vi "Autonomous Independent.vi"   [LabVIEW 2013]
doc: "This VI is called when autonomous begins, and will automatically be terminated when autonomous ends. You can carry out timed or sensor driven robot movement independently without needing to return to the caller."
uses:
  <vilib>/Rock Robotics/WPI/SafetyOutput/WPI_SafetyOutputConfigMenu.ctl
  <vilib>/Rock Robotics/WPI/Solenoid/WPI_SolenoidValue.ctl
  <vilib>/Rock Robotics/WPI/Relay/WPI_RelayValue.ctl
  Robot Global Data.vi
  <vilib>/Rock Robotics/WPI/RobotDrive/WPI_RobotDriveGetSetRefNum.vi
  <vilib>/Rock Robotics/WPI/Solenoid/WPI_SolenoidSetEnum.vi
  <vilib>/Rock Robotics/WPI/RobotDrive/WPI_RobotDriveArcadeDrive_Standard(NoSaturation).vi
  <vilib>/Rock Robotics/WPI/Joystick/WPI_JoystickGetSetRefNum.vi
panel:
  # "Be sure to right-click and choose Data Operations>>Make Current Value default if you want to save the array values with the VI"
types:
  T1 = typedef "WPI_SafetyOutputConfigMenu.ctl" = enum16{"Enable", "Disable"}
  T2 = typedef "WPI_RelayValue.ctl" = enum16{"Off", "On", "Forward", "Reverse"}
  T3 = typedef "WPI_SolenoidValue.ctl" = enum16{"Off", "On", "Forward", "Reverse"}
  T4 = typedef "WPI_JoystickDevRef.ctl" = cluster{"Device":T5}
  T5 = typedef "WPI_JoystickDeviceEnum.ctl" = enum16{"USB 1", "USB 2", "USB 3", "USB 4", "Kinect 1", "Kinect 2"}
  T6 = cluster{"axis 1 (x)":dbl, "axis 2 (y)":dbl, "axis 3 (throttle)":dbl, "axis 4":dbl, "axis 5":dbl, "axis 6":dbl}
  T7 = typedef "WPI_RobotDriveDevRef.ctl" = cluster{"DevStatus":errorcluster, "Motors[]":T8[], "Square Inputs":bool, "Max Output":dbl, "Isochronous":bool}
  T8 = typedef "WPI_MotorControlDeviceRef.ctl" = cluster{"DeviceStatus":errorcluster, "Type":enum16{"PWM", "CAN"}, "PWM":cluster{"Digital Module":T9, "PWM Channel":T10, "DeadBand":T11}, "CAN":cluster{"Device Number":u8, "Control Mode":T12, "Semaphore":T13, "Max Vout":dbl}, "Invert":bool, "TransformRef":T14, "InvTransformRef":T14}
  T9 = typedef "FPGA_TypedefDigitalModule.ctl" = enum16{"Digital Module 1", "Digital Module 2"}
  T10 = typedef "FPGA_DIOPWMChannel.ctl" = enum8{"PWM 1", "PWM 2", "PWM 3", "PWM 4", "PWM 5", "PWM 6", "PWM 7", "PWM 8", "PWM 9", "PWM 10", "Invalid"}
  T11 = typedef "WPI_PWMDeadband.ctl" = cluster{"Name":string, "maxPositivePwm":i32, "minPositivePwm":i32, "centerPwm":i32, "maxNegativePwm":i32, "minNegativePwm":i32, "angularRange":u16}
  T12 = typedef "WPI_CANJaguar_ControlMode.ctl" = enum8{"Percent VBus", "Current", "Speed", "Position", "Voltage"}
  T13 = typedef "Semaphore RefNum" = refnum<k1>
  T14 = typedef "WPI_PWMTransform_ConPane.ctl" = refnum<vi>
  T15 = typedef "WPI_SolenoidDevRef.ctl" = cluster{"DevStatus":errorcluster, "Solenoid Module":T16, "Forward Solenoid Channel":T17, "Reverse Solenoid Channel":T17}
  T16 = typedef "FPGA_TypedefSolenoidModule.ctl" = enum16{"Solenoid Module 1", "Solenoid Module 2"}
  T17 = typedef "WPI_SolenoidChannel.ctl" = enum8{"Solenoid 1", "Solenoid 2", "Solenoid 3", "Solenoid 4", "Solenoid 5", "Solenoid 6", "Solenoid 7", "Solenoid 8", "Invalid"}
  T18 = typedef "WPI_RelayDevRef.ctl" = cluster{"DevStatus":errorcluster, "Relay Channel":T19, "Digital Module":T9, "Relay Direction":T20}
  T19 = typedef "FPGA_DIORelayChannel.ctl" = enum8{"Relay 1", "Relay 2", "Relay 3", "Relay 4", "Relay 5", "Relay 6", "Relay 7", "Relay 8", "Invalid"}
  T20 = typedef "WPI_RelayDirection.ctl" = enum16{"Both directions", "Forward only", "Reverse only"}
  T21 = typedef "WPI_AnalogChannelDevRef.ctl" = cluster{"DevStatus":errorcluster, "Analog Module":T22, "Analog Channel":T23}
  T22 = typedef "FPGA_TypedefAnalogModule.ctl" = enum16{"Analog Module 1", "Analog Module 2"}
  T23 = typedef "FPGA_AIChannel.ctl" = enum8{"AI 1", "AI 2", "AI 3", "AI 4", "AI 5", "AI 6", "AI 7", "AI 8", "Invalid"}
diagram:
  (unwired) "This code sets the toggle rate used by the Periodic Tasks VI.  For autonomous mode we slowly flash the USER1 LED on the cRIO.  Look at the Periodic Tasks VI to see how this global value is used."
  (unwired) "Autonomous sample code is disabled so your robot doesn't unexpectantly run in Autonomous mode.  To enable this code, right-click on the edge of the frame and choose either \"Remove Diagram Disable Structure\" or \"Enable This Subdiagram\". You should only enable one of the samples."
  (unwired) "This function is run in parallel when the autonomous period begins. It will be terminated automatically when the period ends.\n\nNote that all Driver Station inputs are automatically latched and will not change once auto begins."
  # "This tells you the driver position\nand alliance color"
  n1 = call <vilib>:"WPI_DriverStationGet Digital Input.vi"() -> ("Driver Station Digital Input (1-8)"=w4:bool[])  [unwired: 11 out]
  n2 = while {
    stop <- FALSE stop-if-true
    n3 = call <vilib>:"WPI_DriverStationReport Robot Code State.vi"("Autonomous"=TRUE) -> ()  [unwired: 10 in, 1 out]
    n4 = Wait (ms)(milliseconds to wait=u32 20) -> ()  [unwired: 1 out]
  }
  n5 = call <vilib>:"WPI_DriverStationGet Alliance Info.vi"() -> ()  [unwired: 12 out]
  n6 = call <vilib>:"WPI_DriverStationGet Analog Input.vi"() -> ()  [unwired: 12 out]
  n7 = global write "Robot Global Data.vi" "LED toggle rate (ms)"(u32 500 ("LED ms toggle rate")) -> ()
  n8 = Index Array(array=w4) -> (element #1=w2:bool, element #2=w1:bool)  [unwired: 8 in, 6 out]
  n9 = case shown="True" w2 {
    frame False {
    }
    frame True {
      # "Every 20ms, report that we are running autonomous\ncode. Loop will abort the same time as the VI."
      # "Use time and/or sensors to control how the robot drives."
      n10 = call <vilib>:"WPI_JoystickRefNum Registry Get.vi"("refnum name"="Joystick 1") -> ("JoystickDevRef"=w35:T4)  [unwired: 1 in, 9 out]
      n11 = call <vilib>:"WPI_JoystickGet.vi"("JoystickDevRef"=w35) -> ("Axes"=w33:T6)  [unwired: 1 in, 5 out]
      n12 = Unbundle By Name(w33) -> ()  [unwired: 1 out]
      n13 = Cluster To Array(cluster=w33) -> (array=w34:dbl[])
      n14 = call <vilib>:"WPI_RobotDriveRefNum Registry Get.vi"("refnum name"="Left and Right Motors") -> ("error out"=w30:errorcluster, "RobotDriveDevRef"=w29:T7)  [unwired: 9 in]
      n15 = call <vilib>:"SD Write Numeric Array.vi"("Numeric Array"=w34, "Name"="Joystick 1/Axes") -> ()  [unwired: 8 in, 2 out]
      n16 = call <vilib>:"WPI_RobotDriveSafetyConfig.vi"("error in (no error)"=w30, "mode"=WPI_SafetyOutputConfigMenu."Disable", "RobotDriveDevRef"=w29) -> ("error out"=w14:errorcluster, "RobotDriveDevRef"=w15:T7)  [unwired: 7 in]
      n17 = call <vilib>:"WPI_SolenoidRefNum Registry Get.vi"("refnum name"="clamp") -> ("error out"=w18:errorcluster, "SolenoidDevRef"=w19:T15)  [unwired: 9 in]
      n18 = call <vilib>:"WPI_SolenoidRefNum Registry Get.vi"("refnum name"="pickup") -> ("error out"=w16:errorcluster, "SolenoidDevRef"=w17:T15)  [unwired: 9 in]
      n19 = call <vilib>:"WPI_SolenoidRefNum Registry Get.vi"("refnum name"="gear") -> ("error out"=w20:errorcluster, "SolenoidDevRef"=w21:T15)  [unwired: 9 in]
      n20 = call <vilib>:"WPI_SolenoidRefNum Registry Get.vi"("refnum name"="lock") -> ("error out"=w22:errorcluster, "SolenoidDevRef"=w23:T15)  [unwired: 9 in]
      n21 = call <vilib>:"WPI_RelayRefNum Registry Get.vi"("refnum name"="light") -> ("error out"=w8:errorcluster, "RelayDevRef"=w9:T18)  [unwired: 9 in]
      n22 = flat-sequence {
        tunnel: [w123] -> w104
        tunnel: [w122] -> w103
        tunnel: [w121] -> w102
        tunnel: [w120] -> w101
        tunnel: [w119] -> w100
        tunnel: [w118] -> w99
        tunnel: [w117] -> w98
        tunnel: [w116] -> w97
        tunnel: [w115] -> w96
        tunnel: [w114] -> w95
        tunnel: w8 -> [w106]
        tunnel: w9 -> [w107]
        tunnel: w14 -> [w122]
        tunnel: w15 -> [w123]
        tunnel: w16 -> [w124]
        tunnel: w17 -> [w125]
        tunnel: w18 -> [w126]
        tunnel: w19 -> [w127]
        tunnel: w20 -> [w108]
        tunnel: w21 -> [w109]
        tunnel: w22 -> [w110]
        tunnel: w23 -> [w111]
        tunnel: [w139] -> w94
        tunnel: w104 -> [w139]
        tunnel: w103 -> [w138]
        tunnel: [w138] -> w93
        tunnel: w102 -> [w137]
        tunnel: [w137] -> w92
        tunnel: [w136] -> w91
        tunnel: w101 -> [w136]
        tunnel: w100 -> [w135]
        tunnel: [w135] -> w90
        tunnel: [w134] -> w89
        tunnel: w99 -> [w134]
        tunnel: [w133] -> w88
        tunnel: w98 -> [w133]
        tunnel: [w132] -> w87
        tunnel: w97 -> [w132]
        tunnel: [w131] -> w86
        tunnel: w96 -> [w131]
        tunnel: [w130] -> w85
        tunnel: w95 -> [w130]
        tunnel: w94 -> [w154]
        tunnel: w93 -> [w153]
        tunnel: w92 -> [w150]
        tunnel: [w150] -> w84
        tunnel: [w149] -> w83
        tunnel: w91 -> [w149]
        tunnel: w90 -> [w148]
        tunnel: [w148] -> w82
        tunnel: [w147] -> w81
        tunnel: w89 -> [w147]
        tunnel: [w146] -> w80
        tunnel: [w145] -> w79
        tunnel: [w144] -> w78
        tunnel: w88 -> [w144]
        tunnel: [w143] -> w77
        tunnel: w87 -> [w143]
        tunnel: [w142] -> w76
        tunnel: w86 -> [w142]
        tunnel: [w141] -> w75
        tunnel: w85 -> [w141]
        tunnel: w13 -> [w166]
        tunnel: w12 -> [w165]
        tunnel: w84 -> [w164]
        tunnel: [w164] -> w74
        tunnel: [w163] -> w73
        tunnel: w83 -> [w163]
        tunnel: w82 -> [w162]
        tunnel: [w162] -> w72
        tunnel: [w161] -> w71
        tunnel: w81 -> [w161]
        tunnel: w80 -> [w160]
        tunnel: [w160] -> w70
        tunnel: w79 -> [w159]
        tunnel: [w159] -> w69
        tunnel: [w158] -> w68
        tunnel: w78 -> [w158]
        tunnel: [w157] -> w67
        tunnel: w77 -> [w157]
        tunnel: [w156] -> w66
        tunnel: w76 -> [w156]
        tunnel: [w155] -> w65
        tunnel: w75 -> [w155]
        tunnel: w74 -> [w180]
        tunnel: w73 -> [w179]
        tunnel: w72 -> [w186]
        tunnel: [w186] -> w64
        tunnel: [w185] -> w63
        tunnel: w71 -> [w185]
        tunnel: w70 -> [w184]
        tunnel: w69 -> [w183]
        tunnel: [w180] -> w62
        tunnel: [w179] -> w61
        tunnel: [w178] -> w60
        tunnel: w68 -> [w178]
        tunnel: [w177] -> w59
        tunnel: w67 -> [w177]
        tunnel: [w176] -> w58
        tunnel: w66 -> [w176]
        tunnel: [w175] -> w57
        tunnel: w65 -> [w175]
        tunnel: w64 -> [w195]
        tunnel: [w195] -> w56
        tunnel: w63 -> [w194]
        tunnel: [w194] -> w55
        tunnel: w62 -> [w193]
        tunnel: [w193] -> w54
        tunnel: w61 -> [w192]
        tunnel: [w192] -> w53
        tunnel: w60 -> [w191]
        tunnel: [w191] -> w52
        tunnel: w59 -> [w190]
        tunnel: [w190] -> w51
        tunnel: w58 -> [w189]
        tunnel: [w189] -> w50
        tunnel: w57 -> [w188]
        tunnel: [w188] -> w49
        tunnel: w56 -> [w205]
        tunnel: [w205] -> w48
        tunnel: w55 -> [w204]
        tunnel: [w204] -> w47
        tunnel: w54 -> [w203]
        tunnel: [w203] -> w46
        tunnel: w53 -> [w202]
        tunnel: [w202] -> w45
        tunnel: w52 -> [w201]
        tunnel: w51 -> [w200]
        tunnel: w50 -> [w197]
        tunnel: w49 -> [w196]
        tunnel: w48 -> [w209]
        tunnel: [w209] -> w44
        tunnel: w47 -> [w208]
        tunnel: [w208] -> w43
        tunnel: w46 -> [w207]
        tunnel: [w207] -> w42
        tunnel: w45 -> [w206]
        tunnel: [w206] -> w41
        tunnel: w44 -> [w217]
        tunnel: [w217] -> w40
        tunnel: w43 -> [w216]
        tunnel: [w216] -> w39
        tunnel: w42 -> [w214]
        tunnel: w41 -> [w213]
        tunnel: w40 -> [w219]
        tunnel: [w219] -> w37
        tunnel: [w218] -> w38
        tunnel: w39 -> [w218]
        tunnel: w38 -> [w221]
        tunnel: w37 -> [w222]
        frame #0 {
          n23 = call-poly <vilib>:"WPI_SolenoidSet.vi"("error in (no error)"=w126, "Value"=WPI_SolenoidValue."Reverse", "SolenoidDevRef"=w127) -> ("error out"=w114:errorcluster, "SolenoidDevRef"=w115:T15)  [unwired: 7 in]
          n24 = call-poly <vilib>:"WPI_SolenoidSet.vi"("error in (no error)"=w108, "Value"=WPI_SolenoidValue."Forward", "SolenoidDevRef"=w109) -> ("error out"=w118:errorcluster, "SolenoidDevRef"=w119:T15)  [unwired: 7 in]
          n25 = call-poly <vilib>:"WPI_SolenoidSet.vi"("error in (no error)"=w110, "Value"=WPI_SolenoidValue."Forward", "SolenoidDevRef"=w111) -> ("error out"=w120:errorcluster, "SolenoidDevRef"=w121:T15)  [unwired: 7 in]
          n26 = call-poly <vilib>:"WPI_SolenoidSet.vi"("error in (no error)"=w124, "Value"=WPI_SolenoidValue."Reverse", "SolenoidDevRef"=w125) -> ("error out"=w116:errorcluster, "SolenoidDevRef"=w117:T15)  [unwired: 7 in]
          n27 = call <vilib>:"WPI_RelaySet.vi"("error in (no error)"=w106, "RelayValue"=WPI_RelayValue."Forward", "RelayDevRef"=w107) -> ()  [unwired: 7 in, 2 out]
        }
        frame #1 {
          n28 = Wait (ms)(milliseconds to wait=u32 400) -> ()  [unwired: 1 out]
        }
        frame #2 {
          n29 = call-poly <vilib>:"WPI_RobotDriveArcadeDrive.vi"("error in (no error)"=w153, "Y axis value"=0.8, "X axis value"=0.0, "RobotDriveDevRef"=w154) -> ("error out"=w145:errorcluster, "RobotDriveDevRef"=w146:T7)  [unwired: 5 in, 1 out]
        }
        frame #3 {
          n30 = while {
            tunnel: w166 -> [w174]
            tunnel: w165 -> [w173]
            stop <- w171 stop-if-true
            n31 = call <vilib>:"WPI_AnalogChannelGetVoltage.vi"("error in (no error)"=w173, "AIDeviceRef"=w174) -> ("Voltage"=w169:dbl)  [unwired: 7 in, 2 out]
            n32 = Wait (ms)(milliseconds to wait=u32 10) -> ()  [unwired: 1 out]
            n33 = Divide(x=w169, y=0.12) -> (x/y=w170:dbl)
            n34 = Less?(x=w170, y=7.0) -> (x < y?=w171:bool)
          }
        }
        frame #4 {
          # "stop"
          n35 = call-poly <vilib>:"WPI_RobotDriveArcadeDrive.vi"("error in (no error)"=w183, "Y axis value"=0.0, "X axis value"=0.0, "RobotDriveDevRef"=w184) -> ()  [unwired: 5 in, 3 out]
        }
        frame #5 {
          n36 = Wait (ms)(milliseconds to wait=u32 500) -> ()  [unwired: 1 out]
        }
        frame #6 {
          # "let go of ball"
          n37 = call-poly <vilib>:"WPI_SolenoidSet.vi"("error in (no error)"=w196, "Value"=WPI_SolenoidValue."Forward", "SolenoidDevRef"=w197) -> ()  [unwired: 7 in, 2 out]
          n38 = call-poly <vilib>:"WPI_SolenoidSet.vi"("error in (no error)"=w200, "Value"=WPI_SolenoidValue."Forward", "SolenoidDevRef"=w201) -> ()  [unwired: 7 in, 2 out]
        }
        frame #7 {
          # "check for hot goal"
          n39 = while {
            stop <- w212 stop-if-true
            n40 = Wait (ms)(milliseconds to wait=u32 10) -> ()  [unwired: 1 out]
            n41 = call <vilib>:"SD Read Boolean.vi"("Name"="Goal is hot") -> ("Boolean"=w212:bool)  [unwired: 8 in, 2 out]
          }
        }
        frame #8 {
          # "fire"
          n42 = call-poly <vilib>:"WPI_SolenoidSet.vi"("error in (no error)"=w213, "Value"=WPI_SolenoidValue."Reverse", "SolenoidDevRef"=w214) -> ()  [unwired: 7 in, 2 out]
        }
        frame #9 {
          n43 = Wait (ms)(milliseconds to wait=u32 2000) -> ()  [unwired: 1 out]
        }
        frame #10 {
          # "ready for tele"
          n44 = call-poly <vilib>:"WPI_SolenoidSet.vi"("error in (no error)"=w221, "Value"=WPI_SolenoidValue."Reverse", "SolenoidDevRef"=w222) -> ()  [unwired: 7 in, 2 out]
        }
      }
      n45 = call <vilib>:"WPI_AnalogChannelRefNum Registry Get.vi"("refnum name"="sensor") -> ("error out"=w12:errorcluster, "AIDeviceRef"=w13:T21)  [unwired: 9 in]
    }
  }
  n46 = case shown="True" w1 {
    frame False {
    }
    frame True {
      n47 = call <vilib>:"WPI_RobotDriveRefNum Registry Get.vi"("refnum name"="Left and Right Motors") -> ("error out"=w311:errorcluster, "RobotDriveDevRef"=w310:T7)  [unwired: 9 in]
      n48 = call <vilib>:"WPI_RobotDriveSafetyConfig.vi"("error in (no error)"=w311, "mode"=WPI_SafetyOutputConfigMenu."Disable", "RobotDriveDevRef"=w310) -> ("error out"=w293:errorcluster, "RobotDriveDevRef"=w294:T7)  [unwired: 7 in]
      n49 = call <vilib>:"WPI_SolenoidRefNum Registry Get.vi"("refnum name"="clamp") -> ("error out"=w299:errorcluster, "SolenoidDevRef"=w300:T15)  [unwired: 9 in]
      n50 = call <vilib>:"WPI_SolenoidRefNum Registry Get.vi"("refnum name"="pickup") -> ("error out"=w297:errorcluster, "SolenoidDevRef"=w298:T15)  [unwired: 9 in]
      n51 = call <vilib>:"WPI_SolenoidRefNum Registry Get.vi"("refnum name"="gear") -> ("error out"=w301:errorcluster, "SolenoidDevRef"=w302:T15)  [unwired: 9 in]
      n52 = call <vilib>:"WPI_SolenoidRefNum Registry Get.vi"("refnum name"="lock") -> ("error out"=w303:errorcluster, "SolenoidDevRef"=w304:T15)  [unwired: 9 in]
      n53 = flat-sequence {
        tunnel: [w328] -> w295
        tunnel: [w327] -> w292
        tunnel: [w326] -> w288
        tunnel: [w325] -> w283
        tunnel: [w324] -> w282
        tunnel: [w323] -> w273
        tunnel: [w322] -> w261
        tunnel: [w321] -> w257
        tunnel: [w320] -> w253
        tunnel: [w319] -> w249
        tunnel: w293 -> [w327]
        tunnel: w294 -> [w328]
        tunnel: w297 -> [w329]
        tunnel: w298 -> [w330]
        tunnel: w299 -> [w331]
        tunnel: w300 -> [w332]
        tunnel: w301 -> [w313]
        tunnel: w302 -> [w314]
        tunnel: w303 -> [w315]
        tunnel: w304 -> [w316]
        tunnel: [w344] -> w296
        tunnel: w295 -> [w344]
        tunnel: w292 -> [w343]
        tunnel: [w343] -> w291
        tunnel: w288 -> [w342]
        tunnel: [w342] -> w287
        tunnel: [w341] -> w284
        tunnel: w283 -> [w341]
        tunnel: w282 -> [w340]
        tunnel: [w340] -> w281
        tunnel: [w339] -> w274
        tunnel: w273 -> [w339]
        tunnel: [w338] -> w262
        tunnel: w261 -> [w338]
        tunnel: [w337] -> w258
        tunnel: w257 -> [w337]
        tunnel: [w336] -> w254
        tunnel: w253 -> [w336]
        tunnel: [w335] -> w250
        tunnel: w249 -> [w335]
        tunnel: w296 -> [w359]
        tunnel: w291 -> [w358]
        tunnel: w287 -> [w355]
        tunnel: [w355] -> w286
        tunnel: [w354] -> w285
        tunnel: w284 -> [w354]
        tunnel: w281 -> [w353]
        tunnel: [w353] -> w280
        tunnel: [w352] -> w275
        tunnel: w274 -> [w352]
        tunnel: [w351] -> w272
        tunnel: [w350] -> w271
        tunnel: [w349] -> w263
        tunnel: w262 -> [w349]
        tunnel: [w348] -> w259
        tunnel: w258 -> [w348]
        tunnel: [w347] -> w255
        tunnel: w254 -> [w347]
        tunnel: [w346] -> w251
        tunnel: w250 -> [w346]
        tunnel: w290 -> [w361]
        tunnel: w289 -> [w360]
        tunnel: w286 -> [w371]
        tunnel: [w371] -> w270
        tunnel: [w370] -> w269
        tunnel: w285 -> [w370]
        tunnel: w280 -> [w369]
        tunnel: [w369] -> w268
        tunnel: [w368] -> w267
        tunnel: w275 -> [w368]
        tunnel: w272 -> [w367]
        tunnel: [w367] -> w266
        tunnel: w271 -> [w366]
        tunnel: [w366] -> w265
        tunnel: [w365] -> w264
        tunnel: w263 -> [w365]
        tunnel: [w364] -> w260
        tunnel: w259 -> [w364]
        tunnel: [w363] -> w256
        tunnel: w255 -> [w363]
        tunnel: [w362] -> w252
        tunnel: w251 -> [w362]
        tunnel: w270 -> [w391]
        tunnel: [w391] -> w248
        tunnel: w269 -> [w390]
        tunnel: [w390] -> w246
        tunnel: w268 -> [w389]
        tunnel: [w389] -> w244
        tunnel: w267 -> [w388]
        tunnel: [w388] -> w242
        tunnel: w266 -> [w385]
        tunnel: w265 -> [w384]
        tunnel: w264 -> [w381]
        tunnel: w260 -> [w380]
        tunnel: w256 -> [w383]
        tunnel: w252 -> [w382]
        tunnel: [w383] -> w240
        tunnel: [w382] -> w238
        tunnel: [w381] -> w236
        tunnel: [w380] -> w234
        tunnel: w248 -> [w400]
        tunnel: [w400] -> w247
        tunnel: w246 -> [w399]
        tunnel: [w399] -> w245
        tunnel: w244 -> [w398]
        tunnel: [w398] -> w243
        tunnel: w242 -> [w397]
        tunnel: [w397] -> w241
        tunnel: w240 -> [w396]
        tunnel: [w396] -> w239
        tunnel: w238 -> [w395]
        tunnel: [w395] -> w237
        tunnel: w236 -> [w394]
        tunnel: [w394] -> w235
        tunnel: w234 -> [w393]
        tunnel: [w393] -> w233
        tunnel: w247 -> [w410]
        tunnel: [w410] -> w232
        tunnel: w245 -> [w409]
        tunnel: [w409] -> w230
        tunnel: w243 -> [w408]
        tunnel: [w408] -> w228
        tunnel: w241 -> [w407]
        tunnel: [w407] -> w226
        tunnel: w239 -> [w404]
        tunnel: w237 -> [w403]
        tunnel: w235 -> [w402]
        tunnel: w233 -> [w401]
        tunnel: w232 -> [w415]
        tunnel: [w415] -> w231
        tunnel: w230 -> [w414]
        tunnel: [w414] -> w229
        tunnel: w228 -> [w413]
        tunnel: [w413] -> w227
        tunnel: w226 -> [w412]
        tunnel: [w412] -> w225
        tunnel: w231 -> [w419]
        tunnel: w229 -> [w418]
        tunnel: w227 -> [w417]
        tunnel: [w417] -> w279
        tunnel: [w416] -> w276
        tunnel: w225 -> [w416]
        tunnel: w279 -> [w422]
        tunnel: [w422] -> w278
        tunnel: [w421] -> w277
        tunnel: w276 -> [w421]
        tunnel: w277 -> [w424]
        tunnel: w278 -> [w425]
        frame #0 {
          n54 = call-poly <vilib>:"WPI_SolenoidSet.vi"("error in (no error)"=w315, "Value"=WPI_SolenoidValue."Forward", "SolenoidDevRef"=w316) -> ("error out"=w325:errorcluster, "SolenoidDevRef"=w326:T15)  [unwired: 7 in]
          n55 = call-poly <vilib>:"WPI_SolenoidSet.vi"("error in (no error)"=w313, "Value"=WPI_SolenoidValue."Forward", "SolenoidDevRef"=w314) -> ("error out"=w323:errorcluster, "SolenoidDevRef"=w324:T15)  [unwired: 7 in]
          n56 = call-poly <vilib>:"WPI_SolenoidSet.vi"("error in (no error)"=w331, "Value"=WPI_SolenoidValue."Reverse", "SolenoidDevRef"=w332) -> ("error out"=w321:errorcluster, "SolenoidDevRef"=w322:T15)  [unwired: 7 in]
          n57 = call-poly <vilib>:"WPI_SolenoidSet.vi"("error in (no error)"=w329, "Value"=WPI_SolenoidValue."Reverse", "SolenoidDevRef"=w330) -> ("error out"=w319:errorcluster, "SolenoidDevRef"=w320:T15)  [unwired: 7 in]
        }
        frame #1 {
          n58 = Wait (ms)(milliseconds to wait=u32 400) -> ()  [unwired: 1 out]
        }
        frame #2 {
          n59 = call-poly <vilib>:"WPI_RobotDriveArcadeDrive.vi"("error in (no error)"=w358, "Y axis value"=0.8, "X axis value"=0.0, "RobotDriveDevRef"=w359) -> ("error out"=w350:errorcluster, "RobotDriveDevRef"=w351:T7)  [unwired: 5 in, 1 out]
        }
        frame #3 {
          n60 = while {
            tunnel: w361 -> [w379]
            tunnel: w360 -> [w378]
            stop <- w376 stop-if-true
            n61 = call <vilib>:"WPI_AnalogChannelGetVoltage.vi"("error in (no error)"=w378, "AIDeviceRef"=w379) -> ("Voltage"=w374:dbl)  [unwired: 7 in, 2 out]
            n62 = Wait (ms)(milliseconds to wait=u32 10) -> ()  [unwired: 1 out]
            n63 = Divide(x=w374, y=0.12) -> (x/y=w375:dbl)
            n64 = Less?(x=w375, y=7.0) -> (x < y?=w376:bool)
          }
        }
        frame #4 {
          # "stop"
          n65 = call-poly <vilib>:"WPI_RobotDriveArcadeDrive.vi"("error in (no error)"=w384, "Y axis value"=0.0, "X axis value"=0.0, "RobotDriveDevRef"=w385) -> ()  [unwired: 5 in, 3 out]
        }
        frame #5 {
          n66 = Wait (ms)(milliseconds to wait=u32 500) -> ()  [unwired: 1 out]
        }
        frame #6 {
          # "no grip on ball"
          n67 = call-poly <vilib>:"WPI_SolenoidSet.vi"("error in (no error)"=w401, "Value"=WPI_SolenoidValue."Forward", "SolenoidDevRef"=w402) -> ()  [unwired: 7 in, 2 out]
          n68 = call-poly <vilib>:"WPI_SolenoidSet.vi"("error in (no error)"=w403, "Value"=WPI_SolenoidValue."Forward", "SolenoidDevRef"=w404) -> ()  [unwired: 7 in, 2 out]
        }
        frame #7 {
          n69 = Wait (ms)(milliseconds to wait=u32 750) -> ()  [unwired: 1 out]
        }
        frame #8 {
          # "fire"
          n70 = call-poly <vilib>:"WPI_SolenoidSet.vi"("error in (no error)"=w418, "Value"=WPI_SolenoidValue."Reverse", "SolenoidDevRef"=w419) -> ()  [unwired: 7 in, 2 out]
        }
        frame #9 {
          n71 = Wait (ms)(milliseconds to wait=u32 2000) -> ()  [unwired: 1 out]
        }
        frame #10 {
          # "ready for tele"
          n72 = call-poly <vilib>:"WPI_SolenoidSet.vi"("error in (no error)"=w424, "Value"=WPI_SolenoidValue."Reverse", "SolenoidDevRef"=w425) -> ()  [unwired: 7 in, 2 out]
        }
      }
      n73 = call <vilib>:"WPI_AnalogChannelRefNum Registry Get.vi"("refnum name"="sensor") -> ("error out"=w289:errorcluster, "AIDeviceRef"=w290:T21)  [unwired: 9 in]
    }
  }
